vi "testcambienhuong.vi"() -> (2 "yawangle":dbl)   [LabVIEW 2019]
uses:
  <vilib>/myRIO/Instrument Drivers/Onboard IO/I2C/typedefs/I2C User Configuration.ctl
  <vilib>/myRIO/Instrument Drivers/Onboard IO/I2C/typedefs/I2C Transfer Rate.ctl
  <vilib>/Platform/TimedLoop/XDataNode/timing_clust.ctl
  <vilib>/Platform/TimedLoop/XDataNode/nitl_modes.ctl
  <vilib>/Platform/TimedLoop/XDataNode/wakeup.ctl
  <vilib>/myRIO/Instrument Drivers/Onboard IO/I2C/typedefs/I2C Reference.ctl
  <vilib>/myRIO/Common/Instrument Driver Framework/Utilities/typedefs/myRIO Generic Hardware Reference.ctl
  <vilib>/myRIO/Common/Instrument Driver Framework/Utilities/typedefs/Hardware Version Enum.ctl
  <vilib>/myRIO/Common/Instrument Driver Framework/Utilities/typedefs/myRIO v1.0 Reference.ctl
  <vilib>/myRIO/Common/Instrument Driver Framework/Utilities/typedefs/Generic FPGA Reference.ctl
  <vilib>/myRIO/Common/Instrument Driver Framework/myRIO v1.0/I2C/typedefs/I2C Channels Enum.ctl
  <vilib>/myRIO/Instrument Drivers/Onboard IO/I2C/typedefs/I2C Configuration.ctl
  <vilib>/userDefined/High Color/nirio_resource_hc.ctl
  <vilib>/myRIO/Common/Instrument Driver Framework/myRIO v1.0/I2C/vis/myRIO v1.1 Open I2C.vi
  <vilib>/myRIO/Common/Instrument Driver Framework/Utilities/vis/Validate Channels.vi
  <vilib>/myRIO/Common/Instrument Driver Framework/myRIO v1.0/I2C/vis/myRIO v1.0 Reserve I2C.vi
  <vilib>/myRIO/Common/Instrument Driver Framework/myRIO v1.0/UART/vis/myRIO v1.0 Close UART.vi
  <vilib>/myRIO/Common/Instrument Driver Framework/myRIO v1.0/I2C/vis/myRIO v1.0 Build MUX Configuration I2C.vi
  <vilib>/myRIO/Common/Instrument Driver Framework/myRIO v1.0/Resource Manager/vis/myRIO v1.0 Reserve Channel List.vi
  <vilib>/myRIO/Common/Instrument Driver Framework/myRIO v1.0/Resource Manager/vis/myRIO v1.0 Create Configuration List.vi
  <vilib>/myRIO/Common/Instrument Driver Framework/myRIO v1.0/Resource Manager/vis/myRIO v1.0 Reserve Channel.vi
  <vilib>/myRIO/Common/Instrument Driver Framework/myRIO v1.0/Resource Manager/vis/myRIO v1.0 Unreserve Channel.vi
  <vilib>/myRIO/Common/Instrument Driver Framework/myRIO v1.0/Resource Manager/vis/myRIO v1.0 Build Mutex Name.vi
  <vilib>/Utility/VariantDataType/GetNumericInfo.vi
  <vilib>/Utility/error.llb/Error Cluster From Error Code.vi
  <vilib>/myRIO/Common/Instrument Driver Framework/myRIO v1.0/myRIO v1.1 Open.vi
  <vilib>/myRIO/Common/Instrument Driver Framework/Utilities/vis/IO Manager.vi
  <vilib>/myRIO/Common/Instrument Driver Framework/Utilities/vis/Configuration Manager.vi
  <vilib>/myRIO/Common/Instrument Driver Framework/myRIO v1.0/Resource Manager/vis/myRIO v1.0 Configure IO.vi
  <vilib>/myRIO/Common/Instrument Driver Framework/myRIO v1.0/myRIO v1.0 Close.vi
  <vilib>/myRIO/Common/Instrument Driver Framework/myRIO v1.0/I2C/vis/myRIO v1.0 Configure I2C.vi
  <vilib>/myRIO/Common/Instrument Driver Framework/myRIO v1.0/I2C/vis/myRIO v1.0 Write I2C.vi
  <vilib>/myRIO/Common/Instrument Driver Framework/myRIO v1.0/I2C/vis/myRIO v1.0 Read I2C.vi
  <vilib>/myRIO/Common/Instrument Driver Framework/Utilities/vis/FPGA Ref Manager.vi
  <vilib>/myRIO/Common/Instrument Driver Framework/myRIO v1.0/myRIO v1.0 Reset FPGA.vi
  <vilib>/myRIO/Common/Instrument Driver Framework/myRIO v1.0/IRQ/vis/myRIO v1.0 IRQ Info FGV.vi
  <vilib>/myRIO/Common/Instrument Driver Framework/myRIO v1.0/IRQ/vis/myRIO v1.0 Timer IRQ Info FGV.vi
  <vilib>/myRIO/Common/Instrument Driver Framework/myRIO v1.0/IRQ/vis/myRIO v1.0 ISR Agent.vi
  <vilib>/myRIO/Instrument Drivers/Utilities/vis/Reset Index.vi
  <vilib>/myRIO/Common/Instrument Driver Framework/myRIO v1.0/Resource Manager/vis/myRIO v1.0 Block Write Resource Manager.vi
  <vilib>/myRIO/Instrument Drivers/Onboard IO/I2C/vis/myRIO I2C Open.xnode
  <vilib>/platform/TimedLoop/XDataNode/XDataNode.xnode
  <vilib>/myRIO/Instrument Drivers/Onboard IO/I2C/I2C.lvlib
  <vilib>/Platform/TimedLoop/XDataNode/XDNodeRunTimeDep.lvlib
  <vilib>/myRIO/Instrument Drivers/Utilities/Utilities.lvlib
  <vilib>/ptbypt/NI_PtbyPt.lvlib
panel:
  out "offset":dbl
  out "Waveform Chart 2":dbl(graph)
  out "Waveform Chart":dbl(graph)
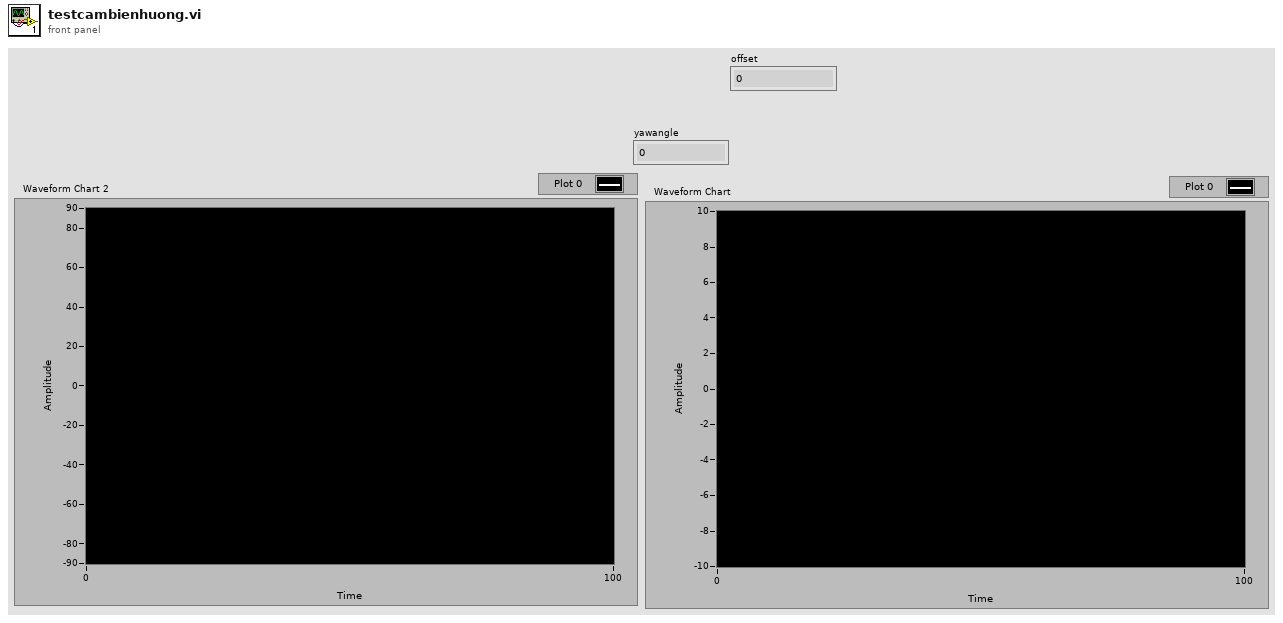
[diagram p1: front panel]
types:
  T1 = typedef "I2C.lvlib/I2C User Configuration.ctl" = cluster{"I2C Transfer Rate":T2}
  T2 = typedef "I2C.lvlib/I2C Transfer Rate.ctl" = enum16{"Standard mode (100 kbps)", "Fast mode (400 kbps)"}
  T3 = typedef "I2C.lvlib/I2C Reference.ctl" = cluster{"myRIO Reference":T4, "I2C Channels Enum":T8, "I2C Configuration":T9}
  T4 = typedef "myRIO Generic Hardware Reference.ctl" = cluster{"myRIO Model":T5, "myRIO Hardware Reference":T6}
  T5 = typedef "Hardware Version Enum.ctl" = enum16{"Unknown", "myRIO-1900", "myRIO-1950", "roboRIO", "NI ELVIS RIO CM", "ELVIS III"}
  T6 = typedef "myRIO v1.0 Reference.ctl" = cluster{"Generic FPGA Reference":T7, "Allow multiple opens":bool}
  T7 = typedef "Generic FPGA Reference.ctl" = refnum<k20>
  T8 = typedef "I2C Channels Enum.ctl" = enum16{"Not Connected", "A/I2C", "B/I2C", "I2C/I2C"}
  T9 = typedef "I2C.lvlib/I2C Configuration.ctl" = cluster{"I2C Transfer Rate":T2}
  T10 = typedef "XDNodeRunTimeDep.lvlib/timing_clust.ctl" = cluster{"Expected End [f-1]":u64, "Actual End [f-1]":u64, "Finished Late? [f-1]":bool, "Expected End [i-1]":u64, "Actual End [i-1]":u64, "Finished Late? [i-1]":bool, "Expected Start [i]":u64, "Actual Start [i]":u64, "Expected Start [f]":u64, "Actual Start [f]":u64, "Source Name":string, "Structure Name":string, "Period":i64, "Deadline":i64, "Offset":i64, "Start":i64, "Priority":i32, "Timeout":i32, "Mode":T11, "Wakeup Reason":T12, "Error":errorcluster, "Source Type":string, "Secondary Source Type":string, "Global End Time":u64, "Global Start Time":u64, "Frame Duration":u64, "Iteration Duration":u64, "Assigned CPU":i32, "I/O Scan Engine Mode":u32}
  T11 = typedef "XDNodeRunTimeDep.lvlib/nitl_modes.ctl" = enum32{"No Change", "Process missed periods, maintain original phase", "Discard missed periods, maintain original phase", "Process missed periods, ignore original phase", "Discard missed periods, ignore original phase"}
  T12 = typedef "XDNodeRunTimeDep.lvlib/wakeup.ctl" = enum32{"Normal", "Aborted", "Asynchronous wakeup", "Timing source error", "Timed loop error", "Timeout"}
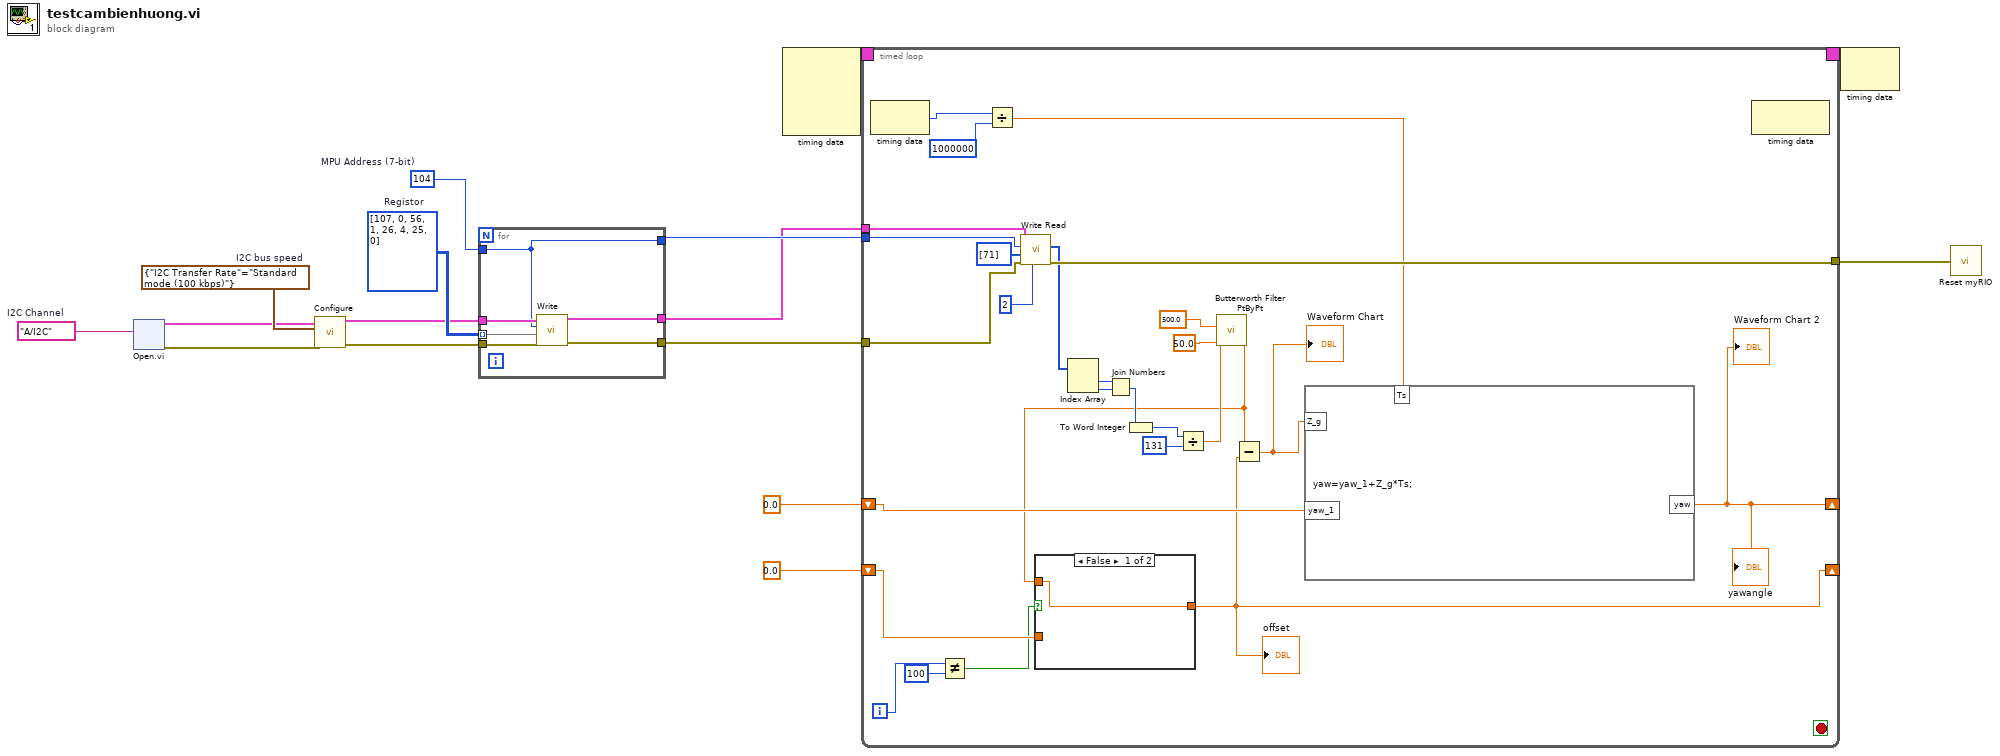
[diagram p0: block diagram]
diagram:
  w11 = u8[][] [[107, 0], [56, 1], [26, 4], [25, 0]]  # Registor
  w8 = u8 104  # MPU Address (7-bit)
  w15 = T1 {"I2C Transfer Rate"=enum."Standard mode (100 kbps)"}  # I2C bus speed
  w16 = tag "A/I2C"  # I2C Channel
  n1 = xnode "Open.vi"("Channel Name"=w16) -> ("error out"=w13:errorcluster, "I2C Ref Out"=w14:T3)  [unwired: 2 in]
  n2 = call <vilib>:"Configure.vi"("error in (no error)"=w13, "I2C User Configuration"=w15, "I2C Ref In"=w14) -> ("error out"=w12:errorcluster, "I2C Ref Out"=w6:T3)  [unwired: 7 in]
  n3 = for {
    tunnel: w12 -> [w22]
    tunnel: w8 -> [w19]
    tunnel: w11 -> [w21] mode=indexing
    tunnel: w6 -> [w20]
    tunnel: [w19] -> w5
    tunnel: [w18] -> w4
    tunnel: [w17] -> w3
    n4 = call <vilib>:"Write.vi"("error in (no error)"=w22, "Bytes to Write"=w21, "Slave Address (7-bit)"=w19, "I2C Ref In"=w20) -> ("error out"=w17:errorcluster, "I2C Ref Out"=w18:T3)  [unwired: 6 in]
  }
  n5 = node-c288() -> (w10:T10)  [unwired: 4 in]
  n6 = timed-loop {
    timing: w10 -> [_]
    timing-out: [_] -> w9
    tunnel: [w47] -> w7
    tunnel: w5 -> [w46]
    tunnel: w4 -> [w45]
    tunnel: w3 -> [w44]
    shift-right: [w29] -> _
    shift-left: 0.0 ("yaw") -> [w34]
    shift-right: [w23] -> _
    shift-left: 0.0 ("Filtered x") -> [w27]
    i -> [w26]
    stop <- _ stop-if-true
    n7 = node-c288() -> (w41:i64)  [unwired: 1 in]
    n8 = Not Equal?(x=w26, y=100) -> (x != y?=w24:bool)
    n9 = Divide(x=w41, y=i64 1000000) -> (x/y=w35:dbl)
    n10 = call <vilib>:"Write Read.vi"("Byte Count"=u32 2, "error in (no error)"=w44, "Bytes to Write"=u8[] [71], "Slave Address (7-bit)"=w46, "I2C Ref In"=w45) -> ("error out"=w47:errorcluster, "Bytes Read"=w43:u8[])  [unwired: 3 in, 1 out]
    n11 = Index Array(array=w43) -> (element #1=w37:u8, element #2=w36:u8)  [unwired: 2 in]
    n12 = Join Numbers(hi=w37, lo=w36) -> ((hi.lo)=w42:u16)
    n13 = To Word Integer(number=w42) -> (16bit integer=w39:i16)
    n14 = Divide(x=w39, y=i16 131) -> (x/y=w33:dbl)
    n15 = call <vilib>:"Butterworth Filter PtByPt.vi"("low cutoff freq: fl"=50.0, "sampling freq: fs"=500.0, "x"=w33) -> ("Filtered x"=w28:dbl)  [unwired: 6 in, 1 out]
    n16 = case shown="False" w24 {
      tunnel: w28 -> [w50 _]
      tunnel: [w50 w51] -> w23
      tunnel: w27 -> [_ w51]
      frame False {
      }
      frame True {
      }
    }
    "offset" <- w23
    n17 = Subtract(x=w28, y=w23) -> (x-y=w30:dbl)
    "Waveform Chart" <- w30
    n18 = formula code="yaw=yaw_1+Z_g*Ts;"("Z_g"=w30, "Ts"=w35, "yaw_1"=w34) -> ("yaw"=w29:dbl)
    "yawangle" <- w29
    "Waveform Chart 2" <- w29
    n19 = node-c288() -> ()  [unwired: 1 in, 1 out]
  }
  n20 = node-c288(w9) -> ()  [unwired: 1 out]
  n21 = call <vilib>:"Reset myRIO.vi"("error in (no error)"=w7) -> ()  [unwired: 10 in, 1 out]
